vi "getAll.vi"(8 "error in (no error)":errorcluster, 11 "Instrument.Oxford VRM in":refnum<class "Instrument.OxfordVRM.lvclass">) -> (0 "error out":errorcluster, 2 "getAll":variant, 3 "Instrument.Oxford VRM out":refnum<class "Instrument.OxfordVRM.lvclass">)   [LabVIEW 2016, in "Instrument.OxfordVRM.lvclass"]
uses:
  Instrument.OxfordVRM.lvclass
  Instrument.OxfordVRM.lvclass/Instrument.OxfordVRM.ctl
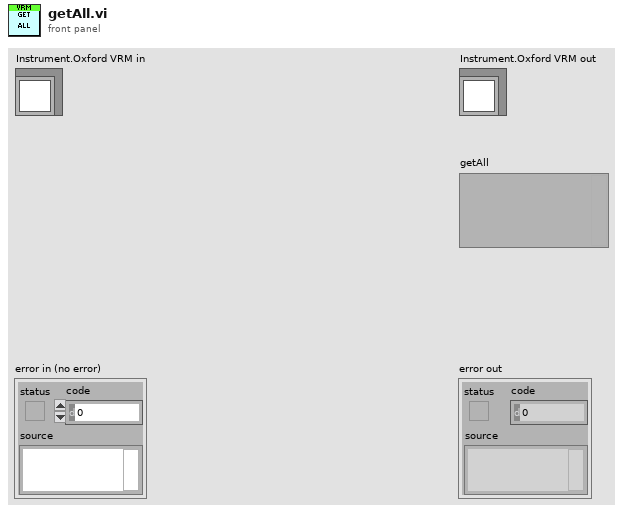
[diagram p1: front panel]
types:
  T1 = typedef "Instrument.OxfordVRM.lvclass/getAll.ctl" = cluster{"Field":dbl[], "Target Field":dbl[], "Target Field Rate":dbl[], "PSU Current":dbl[], "PSU Voltage":dbl[], "Status":string[]}
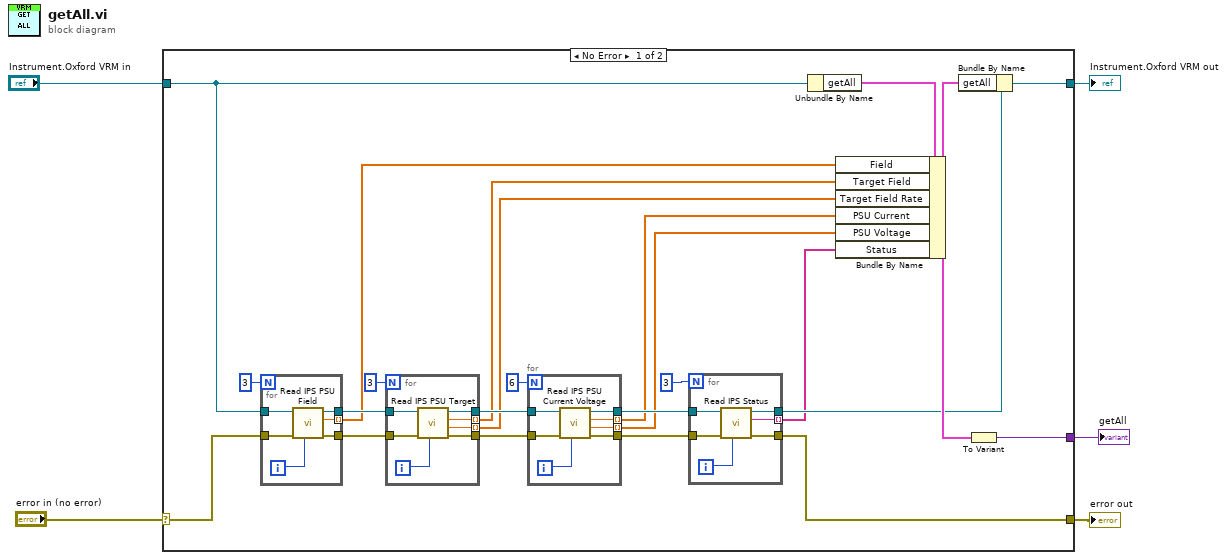
[diagram p0: block diagram]
diagram:
  n1 = case shown="No Error" "error in (no error)" {
    selector: "error in (no error)" -> [w18 w56]
    tunnel: "Instrument.Oxford VRM in" -> [w17 w57]
    tunnel: [w28 w57] -> w4
    tunnel: [w6 w56] -> w2
    tunnel: [w27 _] -> w1
    frame No Error {
      n2 = for {
        N: 3 -> [_]
        tunnel: w17 -> [w41]
        tunnel: w18 -> [w40]
        tunnel: [w38] -> w12 mode=indexing
        tunnel: [w37] -> w20
        tunnel: [w36] -> w21
        i -> [w39]
        n3 = call "Read IPS PSU Field.vi"("Axis"=w39, "error in (no error)"=w40, "Instrument.OxfordVRM in"=w41) -> ("error out"=w37:errorcluster, "Power Supply Field (T)"=w38:dbl, "Instrument.OxfordVRM out"=w36:refnum<class "Instrument.OxfordVRM.lvclass">)  [unwired: 6 in]
      }
      n4 = for {
        N: 3 -> [_]
        tunnel: w21 -> [w48]
        tunnel: w20 -> [w47]
        tunnel: [w45] -> w11 mode=indexing
        tunnel: [w44] -> w10 mode=indexing
        tunnel: [w43] -> w24
        tunnel: [w42] -> w19
        i -> [w46]
        n5 = call "Read IPS PSU Target.vi"("Axis"=w46, "error in (no error)"=w47, "Instrument.OxfordVRM in"=w48) -> ("error out"=w42:errorcluster, "Target Field Rate (T/min)"=w44:dbl, "Target Field (T)"=w45:dbl, "Instrument.OxfordVRM out"=w43:refnum<class "Instrument.OxfordVRM.lvclass">)  [unwired: 5 in]
      }
      n6 = for {
        N: 6 -> [_]
        tunnel: w24 -> [w55]
        tunnel: w19 -> [w54]
        tunnel: [w52] -> w9 mode=indexing
        tunnel: [w51] -> w8 mode=indexing
        tunnel: [w50] -> w16
        tunnel: [w49] -> w14
        i -> [w53]
        n7 = call "Read IPS PSU Current Voltage.vi"("PSU #"=w53, "error in (no error)"=w54, "Instrument.OxfordVRM in"=w55) -> ("error out"=w49:errorcluster, "Voltage (V)"=w51:dbl, "Current (A)"=w52:dbl, "Instrument.OxfordVRM out"=w50:refnum<class "Instrument.OxfordVRM.lvclass">)  [unwired: 5 in]
      }
      n8 = for {
        N: 3 -> [_]
        tunnel: w16 -> [w35]
        tunnel: w14 -> [w34]
        tunnel: [w32] -> w7 mode=indexing
        tunnel: [w31] -> w13
        tunnel: [w30] -> w6
        i -> [w33]
        n9 = call "Read IPS Status.vi"("Axis"=w33, "error in (no error)"=w34, "Instrument.OxfordVRM in"=w35) -> ("error out"=w30:errorcluster, "Status"=w32:string, "Instrument.OxfordVRM out"=w31:refnum<class "Instrument.OxfordVRM.lvclass">)  [unwired: 6 in]
      }
      n10 = Unbundle By Name(w17) -> ("getAll"=w29:T1)
      n11 = Bundle By Name(cluster=w29, "Field"=w12, "Target Field"=w11, "Target Field Rate"=w10, "PSU Current"=w9, "PSU Voltage"=w8, "Status"=w7) -> (w26:T1)
      n12 = Bundle By Name(cluster=w13, "getAll"=w26) -> (w28:refnum<class "Instrument.OxfordVRM.lvclass">)
      n13 = To Variant(anything=w26) -> (Variant=w27:variant)
    }
    frame Error {
    }
  }
  "error out" <- w2
  "Instrument.Oxford VRM out" <- w4
  "getAll" <- w1
